vi "MSScript_Format_SetDAQ.vi"(9 "ValueArray":string[](array[string]), 10 "TagArray":string[](array[string]), 11 "MSScript.lvclass":refnum<class "MSScript.lvclass">) -> (0 "ValueErrorArray":bool[](array[boolean]), 1 "TagErrorArray":bool[](array[boolean]), 2 "ParamErrorArray":bool[](array[boolean]), 3 "Data":variant, 4 "#ofParamError":bool)   [LabVIEW 2018, in "MSScript.lvclass"]
uses:
  MSScript.lvclass
  Ctl/MSEditorParam setDAQ.ctl
  MSScript_Transform_UInt.vi
panel:
  in  "ParamValueType":T1
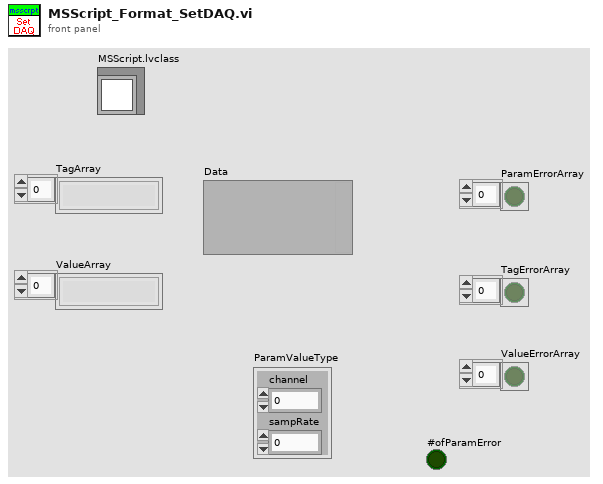
[diagram p1: front panel]
types:
  T1 = typedef "MSEditorParam setDAQ.ctl" = cluster{"channel":u32, "sampRate":u32}
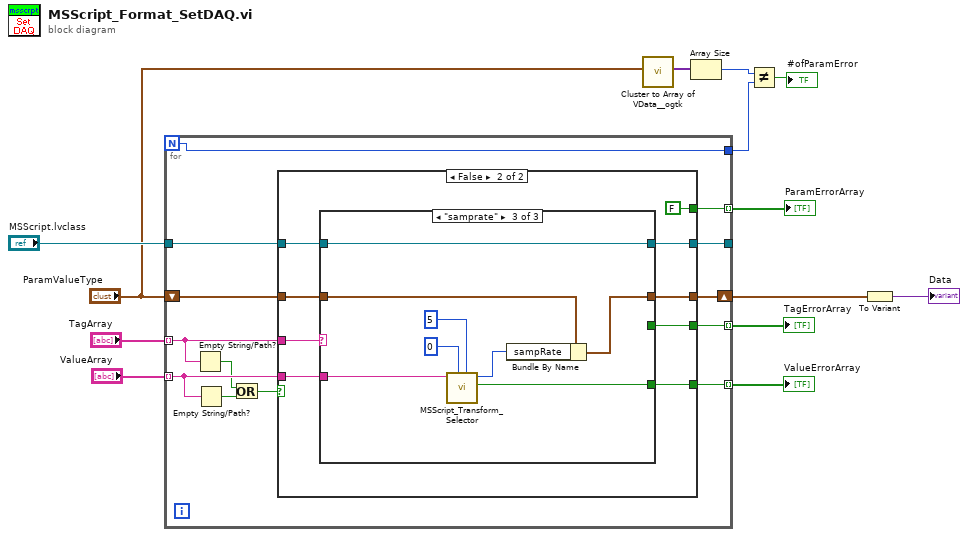
[diagram p0: block diagram]
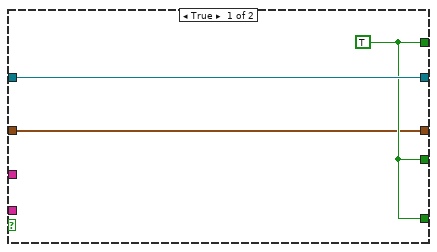
[diagram p2: hidden frame]
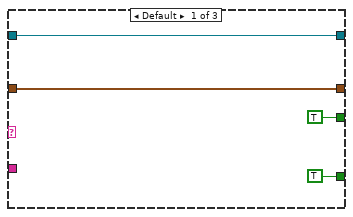
[diagram p3: hidden frame]
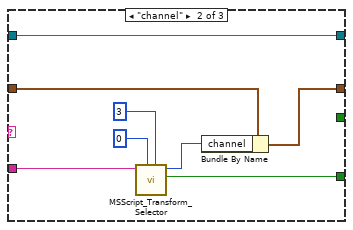
[diagram p4: hidden frame]
diagram:
  n1 = for {
    N -> [w14]
    tunnel: "TagArray" -> [w22] mode=indexing
    tunnel: "ValueArray" -> [w21] mode=indexing
    tunnel: [w26] -> w11 mode=indexing
    tunnel: "MSScript.lvclass" -> [w25]
    tunnel: [w24] -> w10 mode=indexing
    tunnel: [w23] -> _
    tunnel: [w17] -> w9 mode=indexing
    shift-right: [w15] -> w2
    shift-left: "ParamValueType" -> [w16]
    tunnel: [w14] -> w3
    n2 = Empty String/Path?(string/path=w22) -> (empty?=w19:bool)
    n3 = Empty String/Path?(string/path=w21) -> (empty?=w20:bool)
    n4 = Or(x=w19, y=w20) -> (x .or. y?=w18:bool)
    n5 = case shown="False" w18 {
      tunnel: [w28 w35] -> w26
      tunnel: w25 -> [w29 w30]
      tunnel: [w28 w34] -> w24
      tunnel: [w29 w37] -> w23
      tunnel: w22 -> [_ w32]
      tunnel: w21 -> [_ w33]
      tunnel: [w28 FALSE] -> w17
      tunnel: w16 -> [w27 w31]
      tunnel: [w27 w36] -> w15
      frame True {
        w28 = TRUE
      }
      frame False {
        n6 = case shown="\"samprate\"" w32 {
          tunnel: [TRUE _ _] -> w35
          tunnel: w30 -> [w40 w48 w56]
          tunnel: w33 -> [_ w49 w57]
          tunnel: [TRUE ("Value Error?") w50 w58] -> w34
          tunnel: [w40 w48 w56] -> w37
          tunnel: w31 -> [w39 w46 w54]
          tunnel: [w39 w45 w53] -> w36
          frame Default {
          }
          frame "channel" {
            n7 = call-poly "MSScript_Transform_Selector.vi"("upper limit"=u64 3, "lower limit"=u64 0, "string in"=w49) -> ("Value Error?"=w50:bool, "Value Output"=w47:u64)  [unwired: 6 in, 1 out]
            n8 = Bundle By Name(cluster=w46, "channel"=w47) -> (w45:T1)
          }
          frame "samprate" {
            n9 = call-poly "MSScript_Transform_Selector.vi"("upper limit"=u64 5, "lower limit"=u64 0, "string in"=w57) -> ("Value Error?"=w58:bool, "Value Output"=w55:u64)  [unwired: 6 in, 1 out]
            n10 = Bundle By Name(cluster=w54, "sampRate"=w55) -> (w53:T1)
          }
        }
      }
    }
  }
  "TagErrorArray" <- w11
  "ValueErrorArray" <- w10
  "ParamErrorArray" <- w9
  n11 = call <userlib>:"Cluster to Array of VData__ogtk.vi"("Cluster"="ParamValueType") -> ("Array of VData"=w7:variant[])  [unwired: 9 in, 1 out]
  n12 = Array Size(array=w7) -> (size(s)=w6:i32)
  n13 = Not Equal?(x=w6, y=w3) -> (x != y?=→"#ofParamError":bool)
  n14 = To Variant(anything=w2) -> (Variant=→"Data":variant)
